vi "Close pop up window.vi"(6 "Data to send with the notification":variant, 7 "Notifier's name":string, 8 "error in (no error)":errorcluster, 9 "Initialise":bool, 11 "Location":enum16{"Window", "Process"}(ring)) -> (0 "error out":errorcluster, 2 "Stop window's loop (use this to close the window)":bool, 3 "Notification data":variant)   [LabVIEW 2020]
doc: "This VI allows telling a pop up window to close from any location inside a software application.\nOne instance of the VI runs continuously inside the pop up window's main loop waiting for a notification. If the pop up window is not already open, no action is taken.\n\nAny number of instances of this VI can be used throughout the software where you need to tell the pop up window to close.\n\nThe only requirement is that all associated instances of this VI must have the same unique notifier name wired to their input. Any name is allowed.\n\nAdditionally the instance of the VI running inside the pop-up window must be initialised during the first loop iteration by wiring TRUE to its \"Initialise\" input. Its 'Location' input should be set to \"Window\".\n\nAll other instances should have their 'Location' input set to \"Process\".\n\nThe notification can carry data of any type. This can be useful if you want the window to perform a different clean up function depending on which bit of code sent the notification.\n\n\nDeveloped by Theo Koimtzis, 2016"
panel:
  out "created new?":bool
  # "THIS IS A RE-ENTRANT VI"
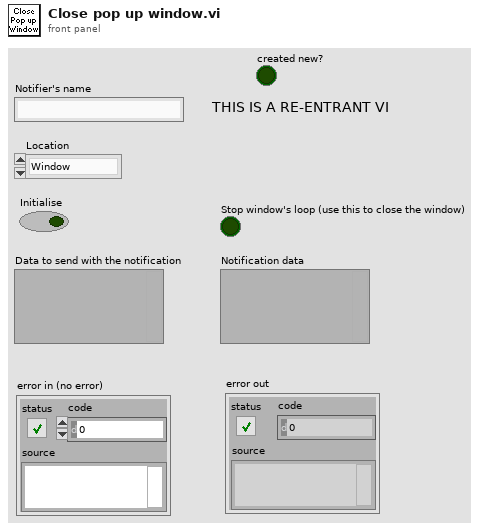
[diagram p1: front panel]
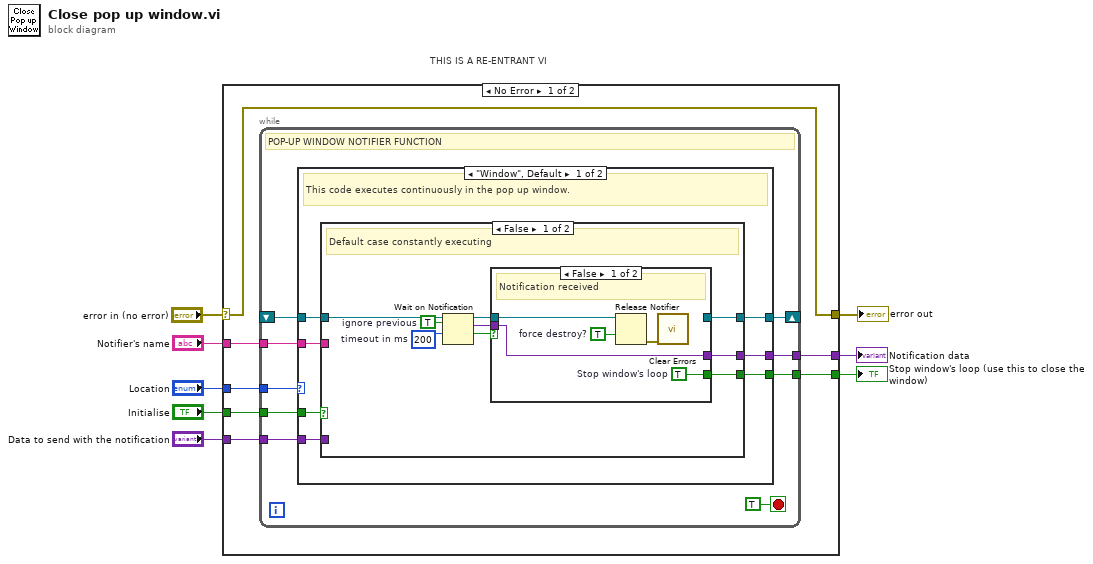
[diagram p0: block diagram]
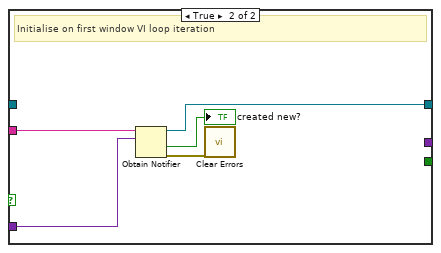
[diagram p3: hidden frame]
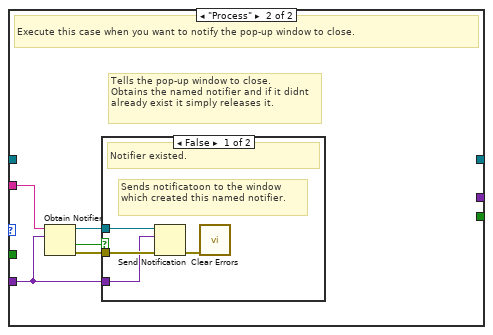
[diagram p4: hidden frame]
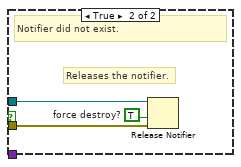
[diagram p5: hidden frame]
diagram:
  # "THIS IS A RE-ENTRANT VI"
  n1 = case shown="No Error" "error in (no error)" {
    selector: "error in (no error)" -> [w9 w64]
    tunnel: [w15 _] -> w8
    tunnel: [w14 _] -> w7
    tunnel: "Initialise" -> [w13 _]
    tunnel: "Location" -> [w12 _]
    tunnel: "Data to send with the notification" -> [w11 _]
    tunnel: "Notifier's name" -> [w10 _]
    tunnel: [w9 w64] -> w1
    frame No Error {
      n2 = while {
        tunnel: w10 -> [w23]
        tunnel: w11 -> [w22]
        tunnel: w12 -> [w21]
        shift-right: [w20] -> _
        shift-left: _ -> [w19]
        tunnel: w13 -> [w18]
        tunnel: [w17] -> w14
        tunnel: [w16] -> w15
        stop <- TRUE stop-if-true
        # "POP-UP WINDOW NOTIFIER FUNCTION"
        n3 = case shown="\"Window\", Default" w21 {
          tunnel: w23 -> [w31 w56]
          tunnel: w22 -> [w30 w52]
          tunnel: [w29 _] -> w20
          tunnel: w19 -> [w27 _]
          tunnel: w18 -> [w28 _]
          tunnel: [w26 _] -> w17
          tunnel: [w25 _] -> w16
          frame "Window", Default {
            # "This code executes continuously in the pop up window."
            n4 = case shown="False" w28 {
              tunnel: w31 -> [_ w51]
              tunnel: w30 -> [_ w50]
              tunnel: [w36 w48] -> w29
              tunnel: w27 -> [w40 _]
              tunnel: [w35 _] -> w26
              tunnel: [w33 _] -> w25
              frame False {
                w32 = TRUE  # ignore previous
                w39 = 200  # timeout in ms
                # "Default case constantly executing"
                n5 = Wait on Notification(notifier=w40, ignore previous (F)=w32, timeout in ms (-1)=w39) -> (notifier out=w37:refnum<notifier>, notification=w34:variant, timed out?=w38:bool)  [unwired: 1 in, 1 out]
                n6 = case shown="False" w38 {
                  tunnel: w37 -> [w43 w46]
                  tunnel: [_ w46] -> w36
                  tunnel: [w42 _] -> w35
                  tunnel: w34 -> [w41 _]
                  tunnel: [w41 _] -> w33
                  frame False {
                    w42 = TRUE  # Stop window's loop
                    w45 = TRUE  # force destroy?
                    # "Notification received"
                    n7 = Release Notifier(notifier=w43, force destroy? (F)=w45) -> (error out=w44:errorcluster)  [unwired: 1 in, 2 out]
                    n8 = call <vilib>:"Clear Errors.vi"("error in (no error)"=w44) -> ()  [unwired: 5 in, 2 out]
                  }
                  frame True {
                    # "No notification received"
                  }
                }
              }
              frame True {
                # "Initialise on first window VI loop iteration"
                n9 = Obtain Notifier(name (unnamed)=w51, notification data type=w50) -> (notifier out=w48:refnum<notifier>, created new?=→"created new?":bool, error out=w49:errorcluster)  [unwired: 2 in]
                n10 = call <vilib>:"Clear Errors.vi"("error in (no error)"=w49) -> ()  [unwired: 5 in, 2 out]
              }
            }
          }
          frame "Process" {
            # "Tells the pop-up window to close.\nObtains the named notifier and if it didnt already exist it simply releases it."
            # "Execute this case when you want to notify the pop-up window to close."
            n11 = Obtain Notifier(name (unnamed)=w56, notification data type=w52) -> (notifier out=w54:refnum<notifier>, created new?=w55:bool, error out=w53:errorcluster)  [unwired: 2 in]
            n12 = case shown="False" w55 {
              tunnel: w54 -> [w60 w63]
              tunnel: w53 -> [w59 w62]
              tunnel: w52 -> [w58 _]
              frame False {
                # "Sends notificatoon to the window which created this named notifier."
                # "Notifier existed."
                n13 = Send Notification(notification=w58, notifier=w60, error in (no error)=w59) -> (error out=w57:errorcluster)  [unwired: 1 out]
                n14 = call <vilib>:"Clear Errors.vi"("error in (no error)"=w57) -> ()  [unwired: 5 in, 2 out]
              }
              frame True {
                w61 = TRUE  # force destroy?
                # "Releases the notifier."
                # "Notifier did not exist."
                n15 = Release Notifier(notifier=w63, force destroy? (F)=w61, error in (no error)=w62) -> ()  [unwired: 3 out]
              }
            }
          }
        }
      }
    }
    frame Error {
    }
  }
  "Stop window's loop (use this to close the window)" <- w7
  "Notification data" <- w8
  "error out" <- w1
